vi "_convertToVariant - Copy.vi"(8 "error in (no error)":errorcluster, 11 "<JSON> 2":string) -> (0 "error out":errorcluster, 3 "Variant":variant)   [LabVIEW 2019]
uses:
  56d81a5c-55a0-4057-82f6-74e2c48c6c43.vi
  5788cce6-90f3-4af3-8d3a-de50f4ee6286.vi
  05839839-6846-41b1-a943-e4a61d359d73.vi
  36c43a05-f3d8-44e6-a819-1d96a9051ce6.vi
  3c089a43-d243-4c10-81d5-6d8e991f8863.vi
  <vilib>/JDP Science/JSONtext/String Subset.vi
  <vilib>/JDP Science/JSONtext/Parsing/Parse Full Path or Item Name.vi
  <vilib>/JDP Science/JSONtext/Next JSON Value.vi
  <vilib>/JDP Science/JSONtext/support/Error Cluster From Code.vi
  <vilib>/JDP Science/JSONtext/Offset/Find Item Locations by Path.vi
  <vilib>/JDP Science/JSONtext/JSON text to Variant.vi
  <vilib>/JDP Science/JSONtext/JSONtext.lvlib
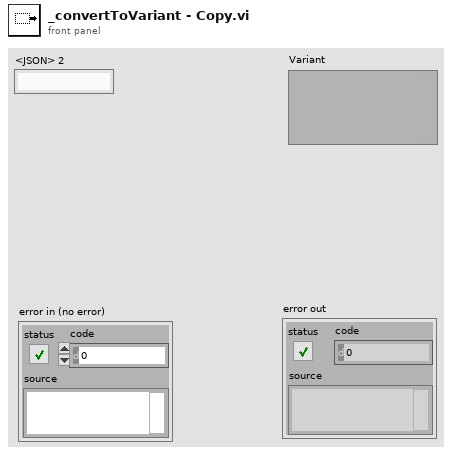
[diagram p1: front panel]
types:
  T1 = typedef "JSONtext.lvlib/JSON Value Type.ctl" = enum16{"Not a JSON Value", "JSON Object", "JSON Array", "String", "Number", "true", "false", "null"}
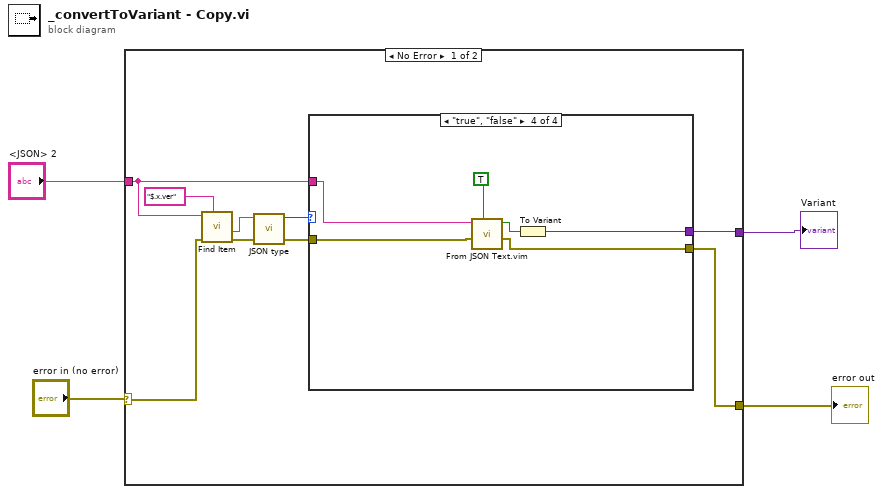
[diagram p0: block diagram]
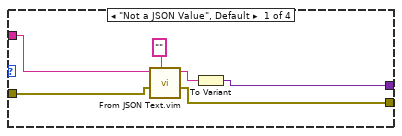
[diagram p2: hidden frame]
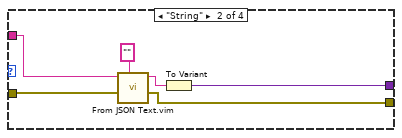
[diagram p3: hidden frame]
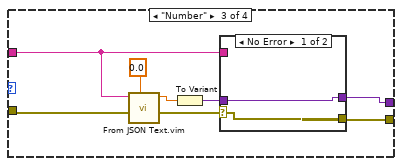
[diagram p4: hidden frame]
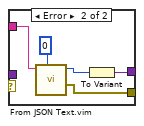
[diagram p5: hidden frame]
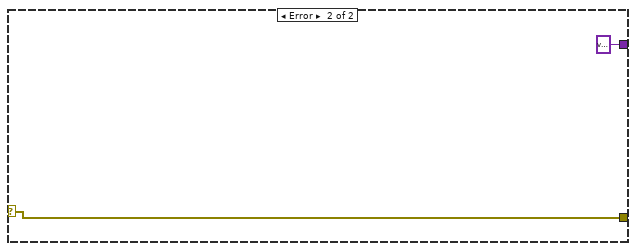
[diagram p6: hidden frame]
diagram:
  n1 = case shown="No Error" "error in (no error)" {
    selector: "error in (no error)" -> [w8 w47]
    tunnel: "<JSON> 2" -> [w9 _]
    tunnel: [w6 variant ("Variant")] -> w2
    tunnel: [w5 w47] -> w1
    frame No Error {
      n2 = call <vilib>:"Find Item.vi"("$Path or Item Name"="$.x.ver", "error in (no error)"=w8, "JSON"=w9) -> ("error out"=w7:errorcluster, "<JSON>"=w11:string)  [unwired: 5 in, 2 out]
      n3 = call <vilib>:"JSON type.vi"("JSON"=w11) -> ("JSON Value Type"=w10:T1)  [unwired: 9 in, 1 out]
      n4 = case shown="\"true\", \"false\"" w10 {
        tunnel: w9 -> [w16 w24 w27 w43]
        tunnel: w7 -> [w15 w23 w31 w40]
        tunnel: [w14 w20 w25 w42] -> w6
        tunnel: [w13 w19 w26 w41] -> w5
        frame "Not a JSON Value", Default {
          n5 = call "From JSON Text.vim"("Data Type and Default Value"="", "error in (no error)"=w15, "JSON"=w16) -> ("error out"=w13:errorcluster, "Data out"=w17:string)  [unwired: 7 in]
          n6 = To Variant(anything=w17) -> (Variant=w14:variant)
        }
        frame "String" {
          n7 = call "From JSON Text.vim"("Data Type and Default Value"="", "error in (no error)"=w23, "JSON"=w24) -> ("error out"=w19:errorcluster, "Data out"=w21:string)  [unwired: 7 in]
          n8 = To Variant(anything=w21) -> (Variant=w20:variant)
        }
        frame "Number" {
          n9 = call "From JSON Text.vim"("Data Type and Default Value"=0.0, "error in (no error)"=w31, "JSON"=w27) -> ("error out"=w29:errorcluster, "Data out"=w32:dbl)  [unwired: 7 in]
          n10 = To Variant(anything=w32) -> (Variant=w28:variant)
          n11 = case shown="No Error" w29 {
            selector: w29 -> [w33 _]
            tunnel: w28 -> [w34 _]
            tunnel: w27 -> [_ w38]
            tunnel: [w33 w37] -> w26
            tunnel: [w34 w35] -> w25
            frame No Error {
            }
            frame Error {
              n12 = call "From JSON Text.vim"("Data Type and Default Value"=u64 0, "JSON"=w38) -> ("error out"=w37:errorcluster, "Data out"=w36:u64)  [unwired: 8 in]
              n13 = To Variant(anything=w36) -> (Variant=w35:variant)
            }
          }
        }
        frame "true", "false" {
          n14 = call "From JSON Text.vim"("Data Type and Default Value"=TRUE, "error in (no error)"=w40, "JSON"=w43) -> ("error out"=w41:errorcluster, "Data out"=w45:bool)  [unwired: 7 in]
          n15 = To Variant(anything=w45) -> (Variant=w42:variant)
        }
      }
    }
    frame Error {
    }
  }
  "error out" <- w1
  "Variant" <- w2
